vi "7 segment in LabVIEW.vi"() -> ()   [LabVIEW 2026]
panel:
  in  "Numeric":dbl
  out "7":bool
  out "6":bool
  out "5":bool
  out "4":bool
  out "3":bool
  out "2":bool
  out "1":bool
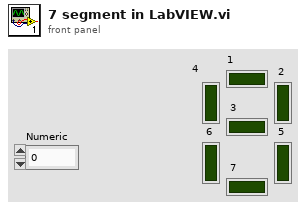
[diagram p1: front panel]
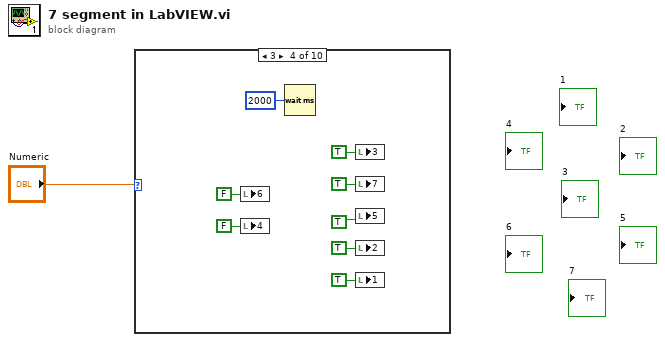
[diagram p0: block diagram]
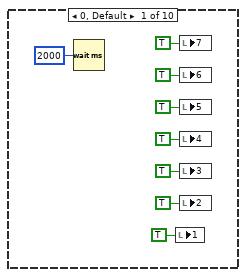
[diagram p2: hidden frame]
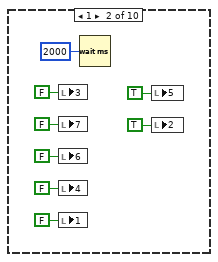
[diagram p3: hidden frame]
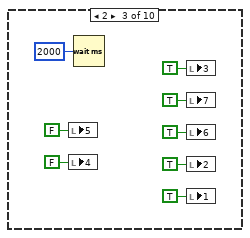
[diagram p4: hidden frame]
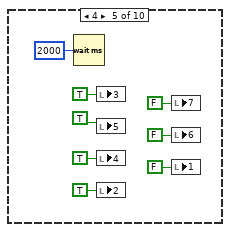
[diagram p5: hidden frame]
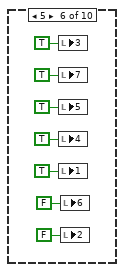
[diagram p6: hidden frame]
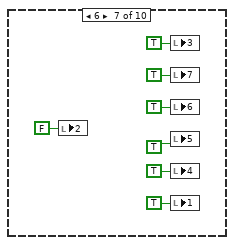
[diagram p7: hidden frame]
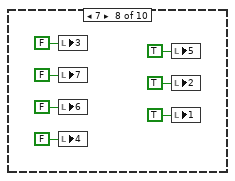
[diagram p8: hidden frame]
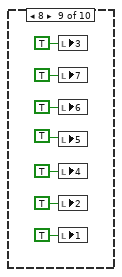
[diagram p9: hidden frame]
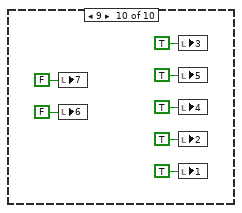
[diagram p10: hidden frame]
diagram:
  n1 = case shown="3" "Numeric" {
    frame 0, Default {
      n2 = Wait (ms)(milliseconds to wait=u32 2000) -> ()  [unwired: 1 out]
      n3 = local write "1"(TRUE ("1")) -> ()
      n4 = local write "7"(TRUE ("7")) -> ()
      n5 = local write "6"(TRUE ("6")) -> ()
      n6 = local write "5"(TRUE ("5")) -> ()
      n7 = local write "4"(TRUE ("4")) -> ()
      n8 = local write "3"(TRUE ("3")) -> ()
      n9 = local write "2"(TRUE ("2")) -> ()
    }
    frame 1 {
      n10 = local write "3"(FALSE ("3")) -> ()
      n11 = local write "7"(FALSE ("7")) -> ()
      n12 = local write "6"(FALSE ("6")) -> ()
      n13 = local write "4"(FALSE ("4")) -> ()
      n14 = local write "1"(FALSE ("1")) -> ()
      n15 = Wait (ms)(milliseconds to wait=u32 2000) -> ()  [unwired: 1 out]
      n16 = local write "5"(TRUE ("5")) -> ()
      n17 = local write "2"(TRUE ("2")) -> ()
    }
    frame 2 {
      n18 = local write "5"(FALSE ("5")) -> ()
      n19 = local write "4"(FALSE ("4")) -> ()
      n20 = Wait (ms)(milliseconds to wait=u32 2000) -> ()  [unwired: 1 out]
      n21 = local write "3"(TRUE ("3")) -> ()
      n22 = local write "7"(TRUE ("7")) -> ()
      n23 = local write "6"(TRUE ("6")) -> ()
      n24 = local write "2"(TRUE ("2")) -> ()
      n25 = local write "1"(TRUE ("1")) -> ()
    }
    frame 3 {
      n26 = local write "6"(FALSE ("6")) -> ()
      n27 = local write "4"(FALSE ("4")) -> ()
      n28 = Wait (ms)(milliseconds to wait=u32 2000) -> ()  [unwired: 1 out]
      n29 = local write "3"(TRUE ("3")) -> ()
      n30 = local write "7"(TRUE ("7")) -> ()
      n31 = local write "5"(TRUE ("5")) -> ()
      n32 = local write "2"(TRUE ("2")) -> ()
      n33 = local write "1"(TRUE ("1")) -> ()
    }
    frame 4 {
      n34 = Wait (ms)(milliseconds to wait=u32 2000) -> ()  [unwired: 1 out]
      n35 = local write "3"(TRUE ("3")) -> ()
      n36 = local write "5"(TRUE ("5")) -> ()
      n37 = local write "4"(TRUE ("4")) -> ()
      n38 = local write "2"(TRUE ("2")) -> ()
      n39 = local write "7"(FALSE ("7")) -> ()
      n40 = local write "6"(FALSE ("6")) -> ()
      n41 = local write "1"(FALSE ("1")) -> ()
    }
    frame 5 {
      n42 = local write "3"(TRUE ("3")) -> ()
      n43 = local write "7"(TRUE ("7")) -> ()
      n44 = local write "5"(TRUE ("5")) -> ()
      n45 = local write "4"(TRUE ("4")) -> ()
      n46 = local write "1"(TRUE ("1")) -> ()
      n47 = local write "6"(FALSE ("6")) -> ()
      n48 = local write "2"(FALSE ("2")) -> ()
    }
    frame 6 {
      n49 = local write "2"(FALSE ("2")) -> ()
      n50 = local write "3"(TRUE ("3")) -> ()
      n51 = local write "7"(TRUE ("7")) -> ()
      n52 = local write "6"(TRUE ("6")) -> ()
      n53 = local write "5"(TRUE ("5")) -> ()
      n54 = local write "4"(TRUE ("4")) -> ()
      n55 = local write "1"(TRUE ("1")) -> ()
    }
    frame 7 {
      n56 = local write "3"(FALSE ("3")) -> ()
      n57 = local write "7"(FALSE ("7")) -> ()
      n58 = local write "6"(FALSE ("6")) -> ()
      n59 = local write "4"(FALSE ("4")) -> ()
      n60 = local write "5"(TRUE ("5")) -> ()
      n61 = local write "2"(TRUE ("2")) -> ()
      n62 = local write "1"(TRUE ("1")) -> ()
    }
    frame 8 {
      n63 = local write "3"(TRUE ("3")) -> ()
      n64 = local write "7"(TRUE ("7")) -> ()
      n65 = local write "6"(TRUE ("6")) -> ()
      n66 = local write "5"(TRUE ("5")) -> ()
      n67 = local write "4"(TRUE ("4")) -> ()
      n68 = local write "2"(TRUE ("2")) -> ()
      n69 = local write "1"(TRUE ("1")) -> ()
    }
    frame 9 {
      n70 = local write "7"(FALSE ("7")) -> ()
      n71 = local write "6"(FALSE ("6")) -> ()
      n72 = local write "3"(TRUE ("3")) -> ()
      n73 = local write "5"(TRUE ("5")) -> ()
      n74 = local write "4"(TRUE ("4")) -> ()
      n75 = local write "2"(TRUE ("2")) -> ()
      n76 = local write "1"(TRUE ("1")) -> ()
    }
  }
